vi "test Add Find Remove Log File.vi"(8 "error in (no error)":errorcluster, 11 "TestCase in":refnum<class "Embedded Data Logger Scripting Unit Tests.lvclass">) -> (0 "error out":errorcluster, 3 "TestCase out":refnum<class "Embedded Data Logger Scripting Unit Tests.lvclass">)   [LabVIEW 2027, in "Embedded Data Logger Scripting Unit Tests.lvclass"]
uses:
  Embedded Data Logger Scripting Unit Tests.lvclass
  C:/Program Files/National Instruments/LabVIEW 2027/vi.lib/NI/VeriStand Custom Device Testing Tools/VeriStandScriptingTestCase/VeriStandScriptingTestCase.lvclass
  <vilib>/NI VeriStand/Custom Device API/Custom Device Item Ref.ctl
  <vilib>/NI/VeriStand Custom Device Testing Tools/VeriStandScriptingTestCase/VeriStandScriptingTestCase.lvclass/VeriStandScriptingTestCase.ctl
  <vilib>/NI/VeriStand Custom Device Testing Tools/VeriStandScriptingTestCase/Read Target.vi
  C:/NetCoreDLL/NationalInstruments.VeriStand.SystemDefinitionAPI.dll
  NetCoreDLL/NationalInstruments.VeriStand.SystemDefinitionAPI.dll
  C:/Program Files/National Instruments/LabVIEW 2027/vi.lib/addons/_JKI Toolkits/VI Tester/TestCase.llb/TestCase.lvclass
  <vilib>/addons/_JKI Toolkits/VI Tester/TestCase.llb/TestCase.lvclass
  <vilib>/NI VeriStand/Custom Device API/Custom Device API.lvlib
  Embedded Data Logger Scripting.lvlib
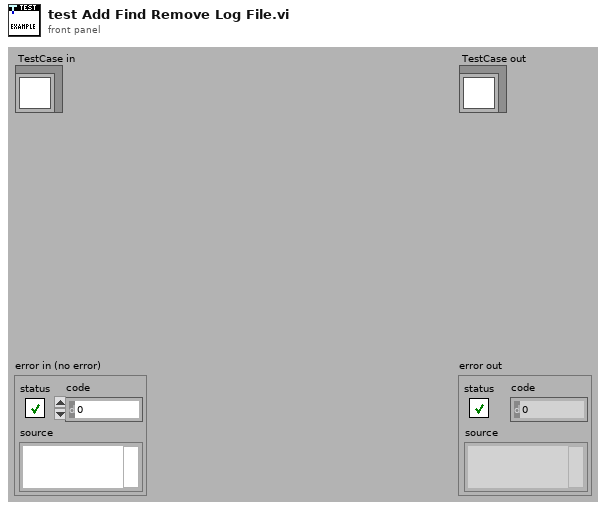
[diagram p1: front panel]
types:
  T1 = typedef "Custom Device API.lvlib/Custom Device Item Ref.ctl" = u64
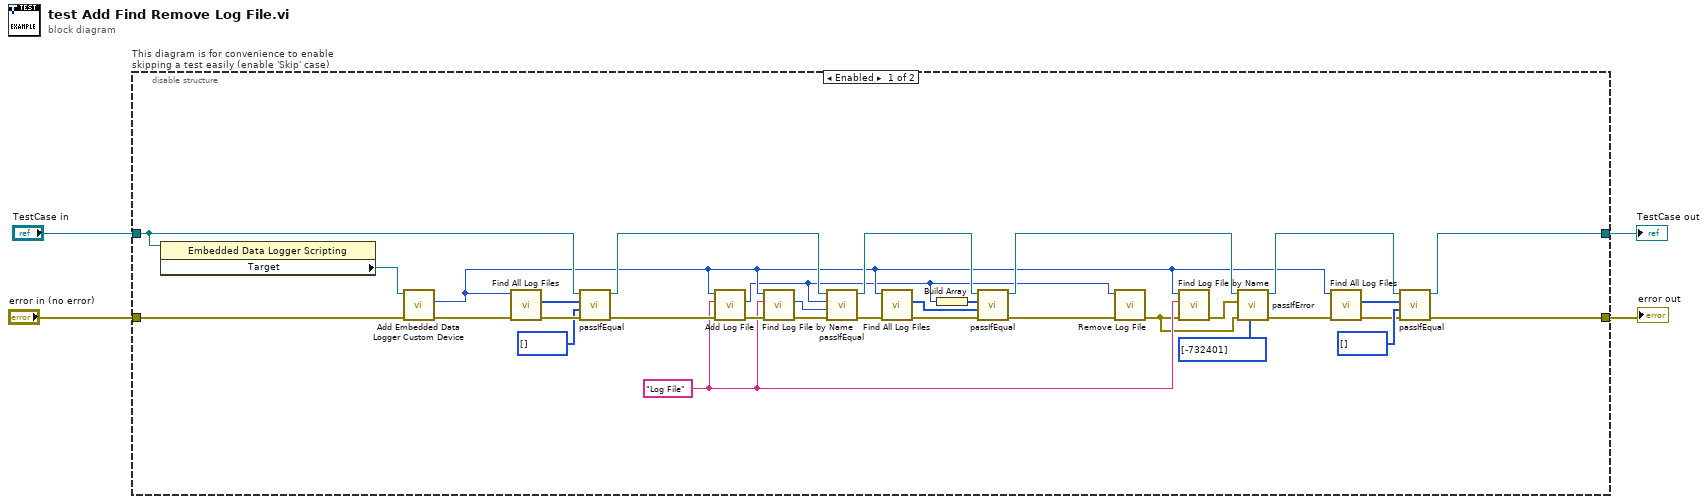
[diagram p0: block diagram]
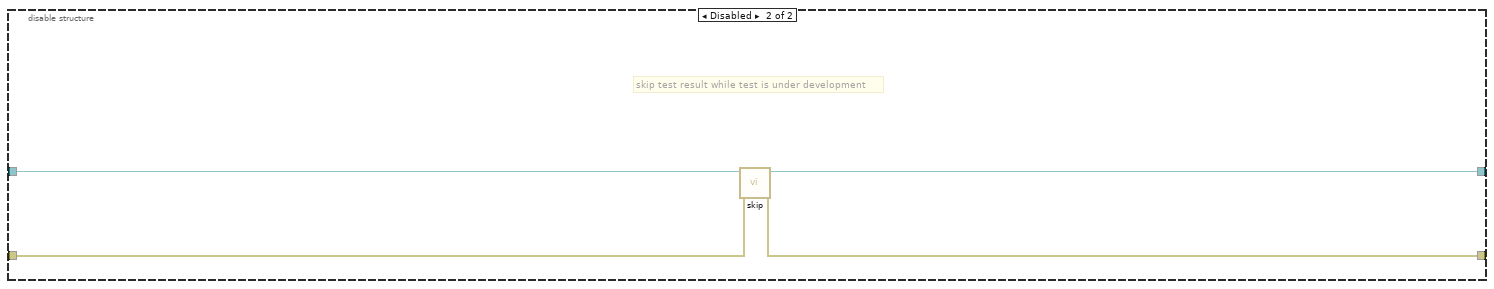
[diagram p2: hidden frame]
diagram:
  n1 = disable-structure "This diagram is for convenience to enable skipping a test easily (enable 'Skip' case)" shown="Enabled" {
    disable-tunnel: "TestCase in" -> [w10 w40]
    disable-tunnel: [w18 w38] -> w1
    disable-tunnel: [w19 w39] -> w3
    disable-tunnel: "error in (no error)" -> [w9 w37]
    frame Enabled {
      w17 = "Log File" ("name")
      n2 = property class="Embedded Data Logger Scripting "(reference=w10) -> ("Target"=w7:refnum<k39>)  [unwired: 1 in, 2 out]
      n3 = call "Add Embedded Data Logger Custom Device.vi"("error in"=w9, "NationalInstruments.VeriStand.SystemDefinitionAPI.Target"=w7) -> ("error out"=w8:errorcluster, "embedded data logger"=w6:T1)  [unwired: 7 in, 1 out]
      n4 = call "Find All Log Files.vi"("error in"=w8, "embedded data logger in"=w6) -> ("error out"=w36:errorcluster, "log files"=w34:T1[])  [unwired: 7 in, 1 out]
      n5 = call-dynamic "passIfEqual.vi"("error in (no error)"=w36, "y"=T1[] [] ("embedded data logger custom devices"), "x"=w34, "TestCase in"=w10) -> ("error out"=w35:errorcluster, "TestCase out"=w26:refnum<class "Embedded Data Logger Scripting Unit Tests.lvclass">)  [unwired: 6 in]
      n6 = call "Add Log File.vi"("error in"=w35, "log file name"=w17, "embedded data logger in"=w6) -> ("error out"=w32:errorcluster, "log file"=w5:T1)  [unwired: 6 in, 1 out]
      n7 = call "Find Log File by Name.vi"("error in"=w32, "log file name"=w17, "embedded data logger in"=w6) -> ("error out"=w29:errorcluster, "log file"=w27:T1)  [unwired: 6 in, 1 out]
      n8 = call-dynamic "passIfEqual.vi"("error in (no error)"=w29, "y"=w27, "x"=w5, "TestCase in"=w26) -> ("error out"=w28:errorcluster, "TestCase out"=w25:refnum<class "Embedded Data Logger Scripting Unit Tests.lvclass">)  [unwired: 6 in]
      n9 = call "Find All Log Files.vi"("error in"=w28, "embedded data logger in"=w6) -> ("error out"=w31:errorcluster, "log files"=w24:T1[])  [unwired: 7 in, 1 out]
      n10 = Build Array(w5) -> (w23:T1[])
      n11 = call-dynamic "passIfEqual.vi"("error in (no error)"=w31, "y"=w24, "x"=w23, "TestCase in"=w25) -> ("error out"=w30:errorcluster, "TestCase out"=w14:refnum<class "Embedded Data Logger Scripting Unit Tests.lvclass">)  [unwired: 6 in]
      n12 = call "Remove Log File.vi"("error in"=w30, "log file"=w5) -> ("error out"=w16:errorcluster)  [unwired: 9 in]
      n13 = call "Find Log File by Name.vi"("error in"=w16, "log file name"=w17, "embedded data logger in"=w6) -> ("error out"=w15:errorcluster)  [unwired: 6 in, 2 out]
      n14 = call-dynamic "passIfError.vi"("passing error codes (default = any error code)"=i32[] [-732401], "error in (no error)"=w16, "error"=w15, "TestCase in"=w14) -> ("error out"=w12:errorcluster, "TestCase out"=w13:refnum<class "Embedded Data Logger Scripting Unit Tests.lvclass">)  [unwired: 6 in]
      n15 = call "Find All Log Files.vi"("error in"=w12, "embedded data logger in"=w6) -> ("error out"=w20:errorcluster, "log files"=w21:T1[])  [unwired: 7 in, 1 out]
      n16 = call-dynamic "passIfEqual.vi"("error in (no error)"=w20, "y"=T1[] [] ("embedded data logger custom devices"), "x"=w21, "TestCase in"=w13) -> ("error out"=w19:errorcluster, "TestCase out"=w18:refnum<class "Embedded Data Logger Scripting Unit Tests.lvclass">)  [unwired: 6 in]
    }
    frame Disabled {
      # "skip test result while test is under development"
      n17 = call <vilib>:"skip.vi"("error in (no error)"=w37, "TestCase in"=w40) -> ("error out"=w39:errorcluster, "TestCase out"=w38:refnum<class "Embedded Data Logger Scripting Unit Tests.lvclass">)  [unwired: 8 in]
    }
  }
  "error out" <- w3
  "TestCase out" <- w1
